vi "ACIR_DCIR_BT3562_testacir.vi"(7 "juste R?":bool, 8 "errin":errorcluster, 9 "chemin de base":path, 10 "section":string="Hioki BT3562", 11 "VISAin":refnum<visa-resource-name>) -> (0 "errout":errorcluster, 1 "OK?":bool, 2 "V":dbl format="%#.3f V", 3 "R":dbl format="%#_6f mOhm", 4 "LogHtml":string[](array[string]), 5 "DataStr":cluster{"Rstr":string, "Vstr":string})   [LabVIEW 2020]
uses:
  <instrlib>/HIOKI BT356X Series/Public/_Initialize/Initialize_serial.vi
  <instrlib>/HIOKI BT356X Series/Public/Action-Status/_Trigger/Init cont.vi
  <instrlib>/HIOKI BT356X Series/Public/Configure/_Trigger/Trigger.vi
  <instrlib>/HIOKI BT356X Series/Public/Configure/_Range/Voltage range.vi
  <instrlib>/HIOKI BT356X Series/Public/Configure/_Range/Resistance range.vi
  <instrlib>/HIOKI BT356X Series/HIOKI BT356X Series.lvlib
panel:
  out "Output Str":string[](array[string])
  out "LogSTD":string
  in  "bin":bool
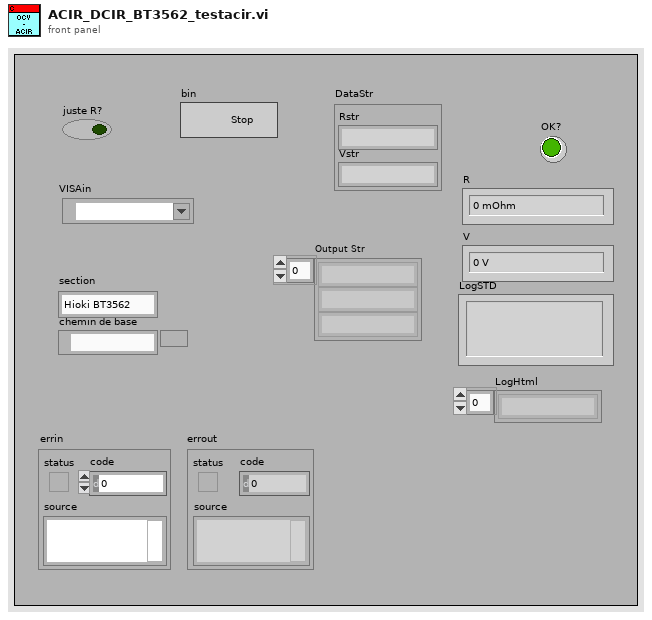
[diagram p1: front panel]
types:
  T1 = enum32{"BT3561A", "BT3562A", "BT3563A", "BT3562", "BT3563", "BT3564", "3561"}
  T2 = cluster{"Timeout":dbl, "Baud":u32, "Vmin":dbl, "Vmax":dbl, "RminMili":dbl, "Rmaxmili":dbl, "Vrange":dbl}
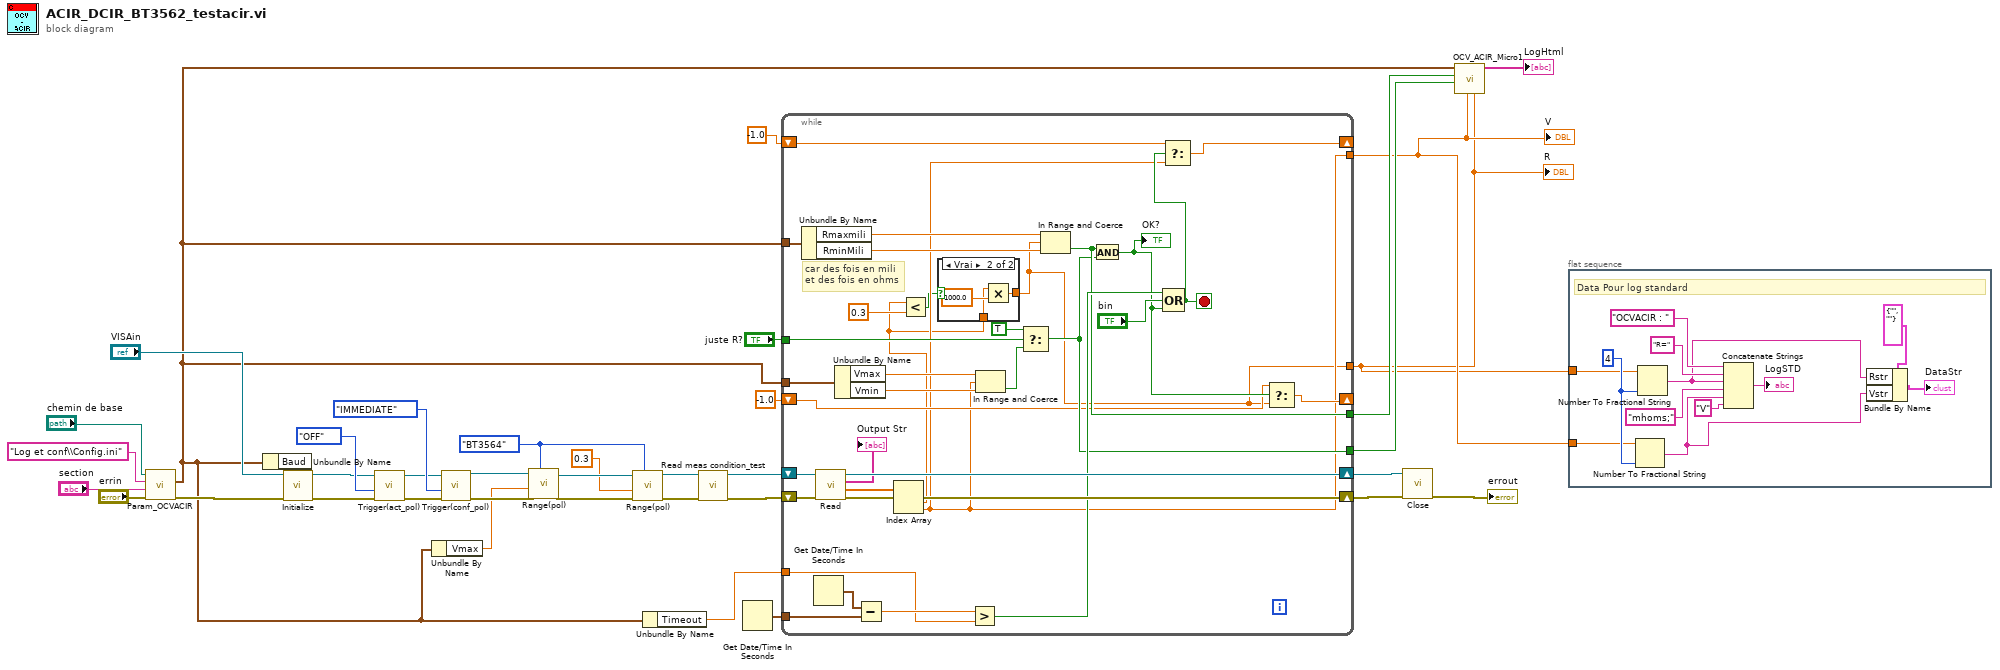
[diagram p0: block diagram]
diagram:
  w5 = T1."BT3564" ("Model")
  n1 = call "Param_OCVACIR.vi"("errin"="errin", "section"="section", "Chaîne"="Log et conf\\Config.ini", "pathin"="chemin de base") -> ("Errout"=w30:errorcluster, "DATA"=w21:T2)  [unwired: 6 in]
  n2 = Unbundle By Name(w21) -> ("Baud"=w10:u32)
  n3 = call-poly <instrlib>:"Initialize.vi"("VISA resource name"="VISAin", "Baud Rate"=w10, "error in (no error)"=w30) -> ("VISA resource name out"=w12:refnum<visa-resource-name>, "error out"=w11:errorcluster)  [unwired: 11 in]
  n4 = call-poly <instrlib>:"Trigger(act_pol).vi"("error in (no error)"=w11, "Do not idle set"=enum16{"ON", "OFF"}."OFF", "VISA session"=w12) -> ("error out"=w15:errorcluster, "dup VISA session"=w14:refnum<visa-resource-name>)  [unwired: 6 in, 1 out]
  n5 = Unbundle By Name(w21) -> ("Vmax"=w1:dbl)
  n6 = call-poly <instrlib>:"Trigger(conf_pol).vi"("error in (no error)"=w15, "Trigger set"=enum16{"IMMEDIATE", "EXTERNAL"}."IMMEDIATE", "VISA session"=w14) -> ("error out"=w8:errorcluster, "dup VISA session"=w9:refnum<visa-resource-name>)  [unwired: 6 in, 1 out]
  n7 = call-poly <instrlib>:"Range(pol).vi"("Model"=w5, "error in (no error)"=w8, "Voltage Range set"=w1, "VISA session"=w9) -> ("error out"=w6:errorcluster, "dup VISA session"=w7:refnum<visa-resource-name>)  [unwired: 5 in, 1 out]
  n8 = call-poly <instrlib>:"Range(pol).vi"("Model"=w5, "error in (no error)"=w6, "Resistance range set"=0.3, "VISA session"=w7) -> ("error out"=w3:errorcluster, "dup VISA session"=w2:refnum<visa-resource-name>)  [unwired: 5 in, 1 out]
  n9 = Unbundle By Name(w21) -> ("Timeout"=w25:dbl)
  n10 = call <instrlib>:"Read meas condition_test.vi"("VISA RefnumIn"=w2, "ErrIn"=w3) -> ("VISA Refnumo"=w34:refnum<visa-resource-name>, "Errout"=w35:errorcluster)  [unwired: 9 in, 3 out]
  n11 = Get Date/Time In Seconds() -> (seconds since 1Jan1904=w33:timestamp)
  n12 = while {
    shift-right: [w69] -> w38
    shift-left: w34 -> [w70]
    shift-right: [w68] -> w37
    shift-left: w35 -> [w71]
    tunnel: w33 -> [w65]
    shift-right: [w61] -> _
    shift-left: -1.0 ("cas faux") -> [w45]
    shift-right: [w60] -> _
    shift-left: -1.0 ("cas faux") -> [w44]
    tunnel: [w49] -> w27
    tunnel: [w59] -> w26
    tunnel: w21 -> [w58]
    tunnel: w25 -> [w55]
    tunnel: w21 -> [w54]
    tunnel: "juste R?" -> [w51]
    tunnel: [w43] -> w18
    tunnel: [w39] -> w17
    stop <- w46 stop-if-true
    # "car des fois en mili \net des fois en ohms"
    n13 = Unbundle By Name(w54) -> ("Rmaxmili"=w53:dbl, "RminMili"=w52:dbl)
    n14 = Get Date/Time In Seconds() -> (seconds since 1Jan1904=w66:timestamp)
    n15 = call <instrlib>:"Read.vi"("error in (no error)"=w71, "VISA session"=w70) -> ("error out"=w68:errorcluster, "Output Val"=w72:dbl[], "Output Str"=→"Output Str":string[], "dup VISA session"=w69:refnum<visa-resource-name>)  [unwired: 6 in]
    n16 = Unbundle By Name(w58) -> ("Vmax"=w57:dbl, "Vmin"=w56:dbl)
    n17 = Subtract(x=w66, y=w65) -> (x-y=w64:dbl)
    n18 = Index Array(array=w72) -> (element #1=w40:dbl, element #2=w43:dbl)  [unwired: 2 in]
    n19 = Less?(x=w40, y=0.3) -> (x < y?=w41:bool)
    n20 = case shown="Vrai" w41 {
      tunnel: w40 -> [w73 w75]
      tunnel: [w73 w74] -> w39
      frame False {
      }
      frame True {
        n21 = Multiply(x=w75, y=1000.0) -> (x*y=w74:dbl)
      }
    }
    n22 = Greater?(x=w64, y=w55) -> (0:w63:bool)
    n23 = In Range and Coerce(upper limit=w57, x=w43, lower limit=w56) -> (In Range?=w50:bool)  [unwired: 1 out]
    n24 = Select(t=TRUE ("cas vrai"), s=w51, f=w50) -> (s? t:f=w49:bool)
    n25 = In Range and Coerce(upper limit=w53, x=w39, lower limit=w52) -> (In Range?=w59:bool)  [unwired: 1 out]
    n26 = And(x=w59, y=w49) -> (x .and. y?=w62:bool)
    "OK?" <- w62
    n27 = Compound Arithmetic op=OR ("Opérateur arithmétique")(w63, "bin", w62) -> (w46:bool)
    n28 = Select(t=w45, s=w46, f=w43) -> (s? t:f=w61:dbl)
    n29 = Select(t=w44, s=w62, f=w39) -> (s? t:f=w60:dbl)
  }
  "R" <- w17
  "V" <- w18
  n30 = call <instrlib>:"Close.vi"("error in (no error)"=w37, "VISA resource name"=w38) -> ("error out"=→"errout":errorcluster)  [unwired: 9 in]
  n31 = call "OCV_ACIR_Micro1.vi"("R"=w17, "V"=w18, "V OK"=w27, "R OK"=w26, "DATA"=w21) -> ("Tableau"=→"LogHtml":string[])  [unwired: 6 in]
  n32 = flat-sequence {
    tunnel: w17 -> [w82]
    tunnel: w18 -> [w81]
    frame #0 {
      w88 = i16 4 ("précision (6)")
      # "Data Pour log standard"
      n33 = Number To Fractional String(number=w81, precision (6)=w88) -> (F-format string=w77:string)  [unwired: 2 in]
      n34 = Number To Fractional String(number=w82, precision (6)=w88) -> (F-format string=w78:string)  [unwired: 2 in]
      n35 = Concatenate Strings("OCVACIR : " ("chaîne"), "R=" ("chaîne"), w78, "mhoms;" ("chaîne"), w77, "V" ("chaîne")) -> (→"LogSTD":string)
      n36 = Bundle By Name(cluster=cluster{"Rstr":string, "Vstr":string} {"Rstr"="", "Vstr"=""} ("DataStr"), "Rstr"=w78, "Vstr"=w77) -> (→"DataStr":cluster{"Rstr":string, "Vstr":string})
    }
  }
